vi "eiptag to table line.vi"(11 "eip tags":T1[](array[typedef])) -> (3 "Item Names":string[][](array[string]))   [LabVIEW 2013, in "EIP Tags editor node.lvclass"]
uses:
  EIP Tags editor node.lvclass
  configuration/EIP Tags Configuration.lvclass
  configuration/eip tag types.ctl
  configuration/eip tag definition.ctl
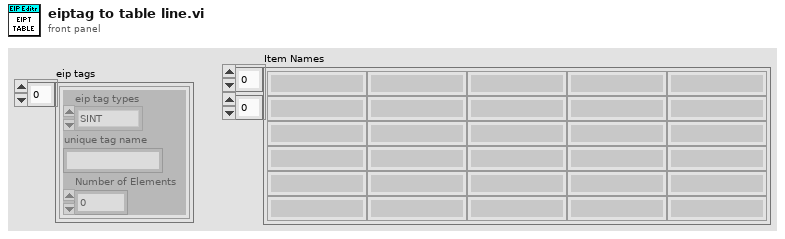
[diagram p1: front panel]
types:
  T1 = typedef "EIP Tags Configuration.lvclass/eip tag definition.ctl" = cluster{"eip tag types":T2, "unique tag name":string, "Number of Elements":u32}
  T2 = typedef "EIP Tags Configuration.lvclass/eip tag types.ctl" = enum16{"SINT", "INT", "DINT", "REAL", "BOOL", "STRING"}
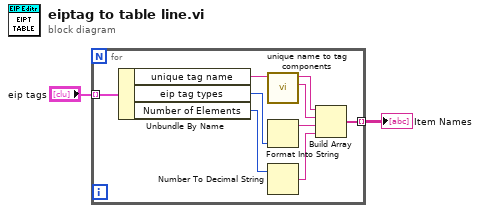
[diagram p0: block diagram]
diagram:
  n1 = for {
    tunnel: "eip tags" -> [w11] mode=indexing
    tunnel: [w8] -> w1 mode=indexing
    n2 = Unbundle By Name(w11) -> ("unique tag name"=w7:string, "eip tag types"=w4:T2, "Number of Elements"=w10:u32)
    n3 = call "unique name to tag components.vi"("unique name"=w7) -> ("Tag Name"=w5:string, "Network Path"=w6:string)  [unwired: 9 in]
    n4 = Format Into String(w4) -> (resulting string=w3:string)  [unwired: 3 in, 1 out]
    n5 = Number To Decimal String(number=w10) -> (decimal integer string=w9:string)  [unwired: 1 in]
    n6 = Build Array(w6, w5, w3, w9) -> (w8:string[])
  }
  "Item Names" <- w1
